vi "XGT 개별읽기 응답프레임.vi"(11 "응답프레임":string="\u000601RSS02021234025678\u0003") -> (1 "숫자변환":i32[](array[numeric]), 2 "에러코드":string, 3 "헥사":string[](array[string]), 7 "블록수 숫자형":i32)   [LabVIEW 2012]
panel:
  # "데이터"
  # "ACK응답 예: 0630 3152 5353 3032 3032 3132 3334 3032 3536 3738 03"
  # "NAK응답 예: 1530 3152 5353 0000 0000 03"
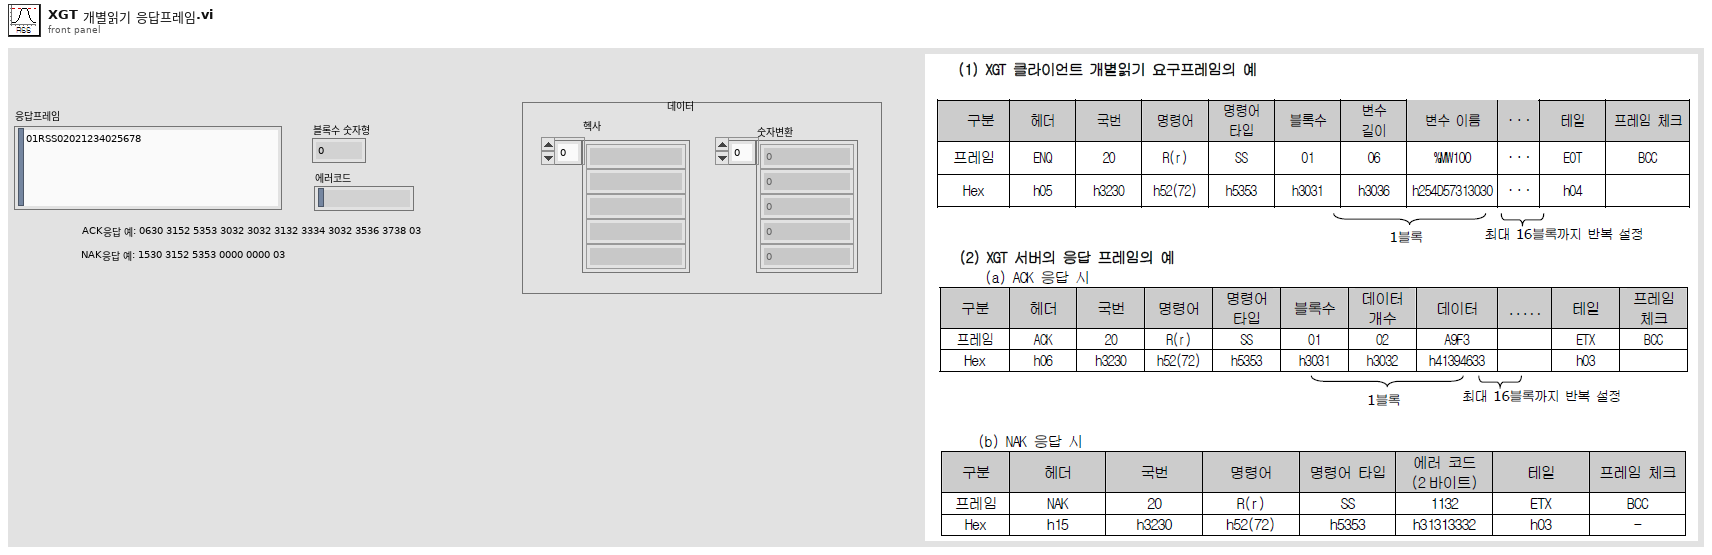
[diagram p1: front panel]
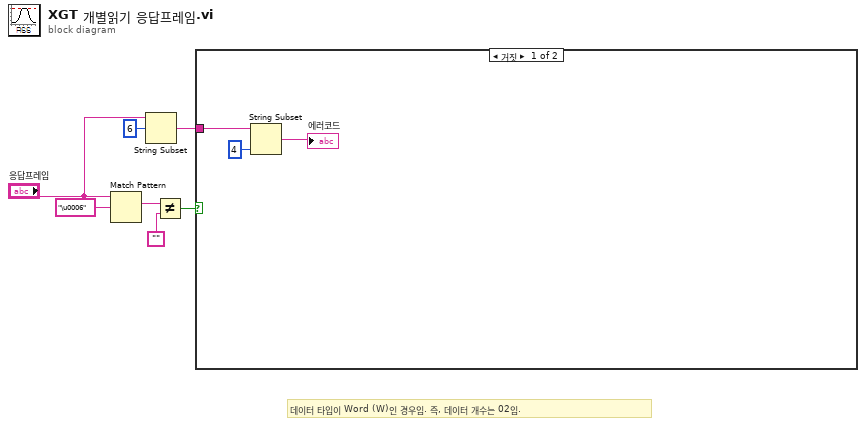
[diagram p0: block diagram]
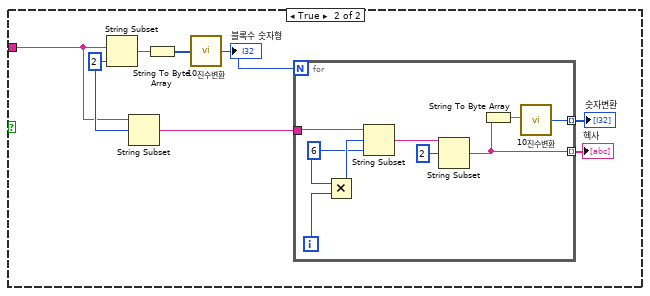
[diagram p2: hidden frame]
diagram:
  # "데이터 타입이 Word (W)인 경우임. 즉, 데이터 개수는 02임."
  n1 = Match Pattern(string="응답프레임", regular expression="\u0006" ("정규식")) -> (match substring=w5:string)  [unwired: 1 in, 3 out]
  n2 = String Subset(string="응답프레임", offset (0)=6 ("오프셋(0)")) -> (substring=w1:string)  [unwired: 1 in]
  n3 = Not Equal?(x=w5, y="") -> (x != y?=w4:bool)
  n4 = case shown="거짓" w4 {
    tunnel: w1 -> [w10 w11]
    frame False {
      n5 = String Subset(string=w10, length (rest)=4 ("길이(나머지)")) -> (substring=→"에러코드":string)  [unwired: 1 in]
    }
    frame True {
      w15 = 2 ("길이(나머지)")
      n6 = String Subset(string=w11, length (rest)=w15) -> (substring=w18:string)  [unwired: 1 in]
      n7 = String Subset(string=w11, offset (0)=w15) -> (substring=w14:string)  [unwired: 1 in]
      n8 = String To Byte Array(string=w18) -> (unsigned byte array=w17:u8[])
      n9 = call "10진수변환.vi"("16진수"=w17) -> ("숫자형"=w16:i32)
      "블록수 숫자형" <- w16
      n10 = for {
        N: w16 -> [_]
        tunnel: w14 -> [w27]
        tunnel: [w20] -> w13 mode=indexing
        tunnel: [w19] -> w12 mode=indexing
        i -> [w25]
        w24 = 6 ("길이(나머지)")
        n11 = Multiply(x=w24, y=w25) -> (x*y=w26:i32)
        n12 = String Subset(string=w27, offset (0)=w26, length (rest)=w24) -> (substring=w23:string)
        n13 = String Subset(string=w23, offset (0)=2 ("오프셋(0)")) -> (substring=w19:string)  [unwired: 1 in]
        n14 = String To Byte Array(string=w19) -> (unsigned byte array=w21:u8[])
        n15 = call "10진수변환.vi"("16진수"=w21) -> ("숫자형"=w20:i32)
      }
      "숫자변환" <- w13
      "헥사" <- w12
    }
  }
